vi "MDPtr ValidateFlattenToString3.vi"() -> ()   [LabVIEW 2017]
uses:
  <vilib>/Utility/High Resolution Relative Seconds.vi
panel:
  out "length 2":i32
  out "Waveform Graph 5":dbl[](graph)
  out "Waveform Graph 4":dbl[](graph)
  out "x-y 2":u32
  out "Waveform Graph 3":dbl[](graph)
  out "Waveform Graph 2":i32[](graph)
  out "Waveform Graph":dbl[](graph)
  out "x-y":u32
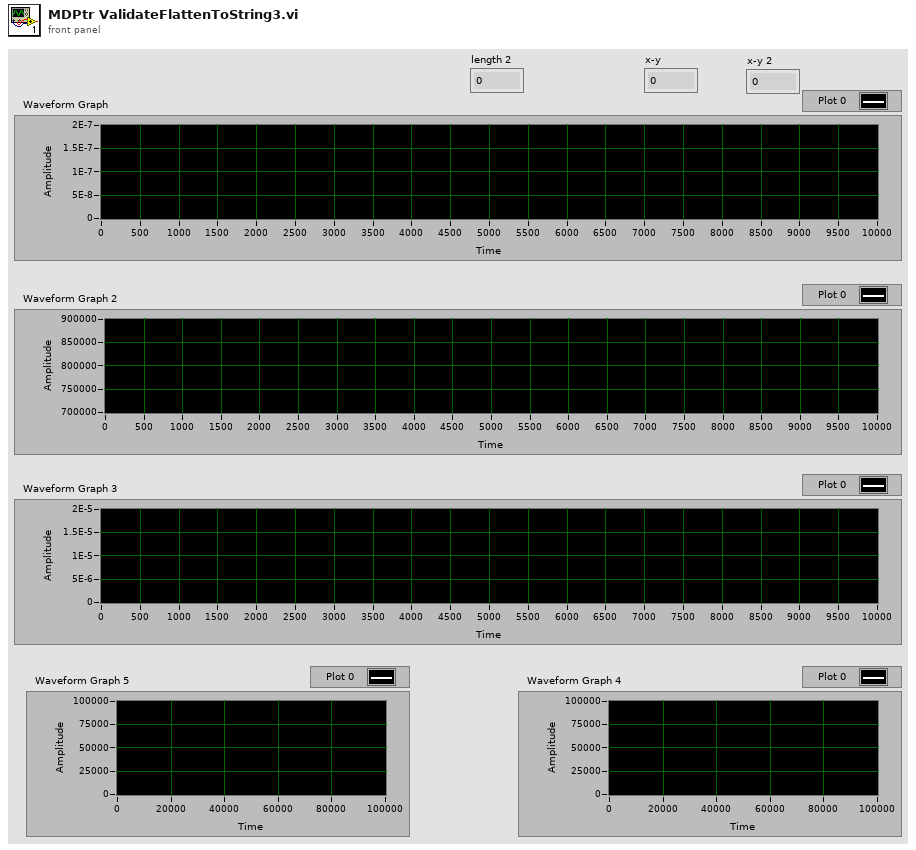
[diagram p1: front panel]
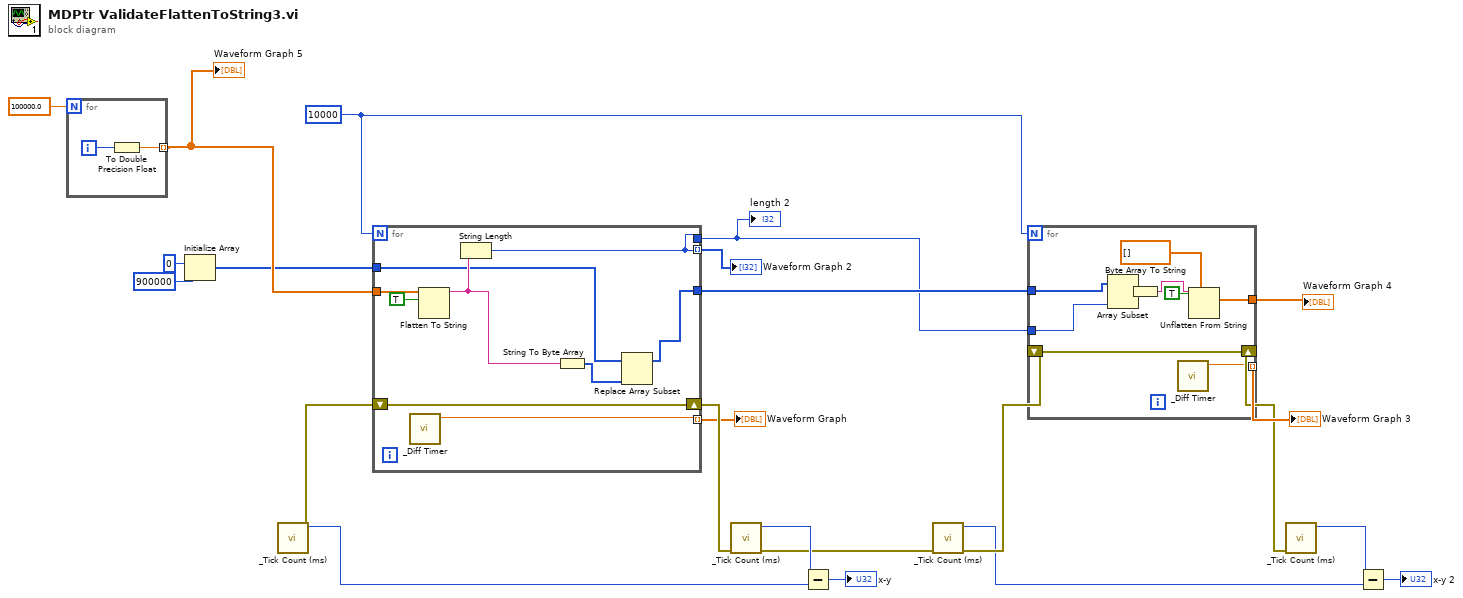
[diagram p0: block diagram]
diagram:
  w8 = 10000
  n1 = for {
    N: 100000.0 ("Fs") -> [_]
    tunnel: [w24] -> w3 mode=indexing
    i -> [w25]
    n2 = To Double Precision Float(number=w25) -> (double precision float=w24:dbl)
  }
  "Waveform Graph 5" <- w3
  n3 = Initialize Array(u8 0 ("element"), 900000 ("dimension size")) -> (w1:u8[])
  n4 = call "_Tick Count (ms).vi"() -> ("error out"=w21:errorcluster, "millisecond timer value"=w22:u32)  [unwired: 10 in]
  n5 = for {
    N: w8 -> [_]
    tunnel: w3 -> [w34]
    tunnel: [w33] -> w18 mode=indexing
    shift-right: [w32] -> w20
    shift-left: w21 -> [w32]
    tunnel: [w31] -> w17 mode=indexing
    tunnel: [w27] -> w9
    tunnel: [w31] -> w5
    tunnel: w1 -> [w26]
    n6 = call "_Diff Timer.vi"() -> ("time diff(s)"=w33:dbl)  [unwired: 10 in, 1 out]
    n7 = Flatten To String(anything=w34, prepend array or string size? (T)=TRUE) -> (data string=w29:string)  [unwired: 2 in, 2 out]
    n8 = String Length(string=w29) -> (length=w31:i32)
    n9 = String To Byte Array(string=w29) -> (unsigned byte array=w28:u8[])
    n10 = Replace Array Subset(array=w26, new element=w28) -> (w27:u8[])  [unwired: 1 in]
  }
  "Waveform Graph" <- w18
  "Waveform Graph 2" <- w17
  "length 2" <- w5
  n11 = call "_Tick Count (ms).vi"("error in (no error)"=w20) -> ("error out"=w10:errorcluster, "millisecond timer value"=w23:u32)  [unwired: 9 in]
  n12 = Subtract(x=w23, y=w22) -> (x-y=→"x-y":u32)
  n13 = call "_Tick Count (ms).vi"("error in (no error)"=w10) -> ("error out"=w13:errorcluster, "millisecond timer value"=w12:u32)  [unwired: 9 in]
  n14 = for {
    N: w8 -> [_]
    tunnel: [w43] -> w16 mode=indexing
    shift-right: [w42] -> w14
    shift-left: w13 -> [w42]
    tunnel: w9 -> [w37]
    tunnel: w5 -> [w41]
    tunnel: [w39] -> w2
    n15 = Array Subset(array=w37, length=w41) -> (w36:u8[])  [unwired: 1 in]
    n16 = Byte Array To String(unsigned byte array=w36) -> (string=w35:string)
    n17 = call "_Diff Timer.vi"() -> ("time diff(s)"=w43:dbl)  [unwired: 10 in, 1 out]
    n18 = Unflatten From String(type=dbl[] [] ("Fs"), binary string=w35, data includes array or string size? (T)=TRUE) -> (value=w39:dbl[])  [unwired: 2 in, 2 out]
  }
  "Waveform Graph 3" <- w16
  "Waveform Graph 4" <- w2
  n19 = call "_Tick Count (ms).vi"("error in (no error)"=w14) -> ("millisecond timer value"=w11:u32)  [unwired: 9 in, 1 out]
  n20 = Subtract(x=w11, y=w12) -> (x-y=→"x-y 2":u32)
